vi "Sort CSV Array.vi"(10 "ListBox Tests in":T1, 11 "New ItemNames":string[](array[string])) -> (2 "Sorted ListBox Tests":T1)   [LabVIEW 2011]
uses:
  Controls/ListBox Test Record.ctl
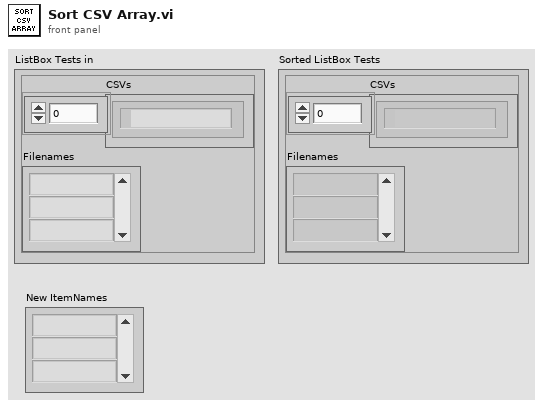
[diagram p1: front panel]
types:
  T1 = typedef "ListBox Test Record.ctl" = cluster{"CSVs":path[], "Filenames":string[]}
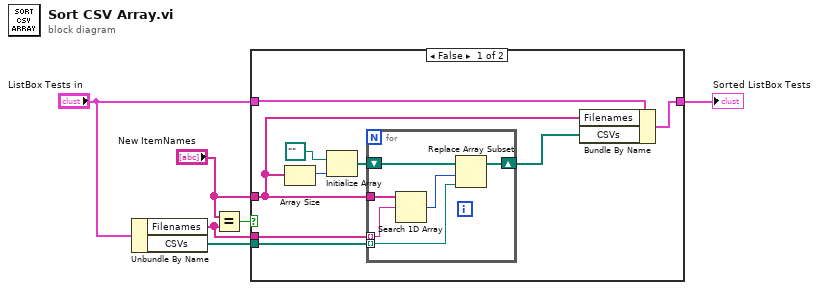
[diagram p0: block diagram]
diagram:
  n1 = Unbundle By Name("ListBox Tests in") -> ("Filenames"=w3:string[], "CSVs"=w1:path[])
  n2 = Equal?(x="New ItemNames", y=w3) -> (x = y?=w6:bool)
  n3 = case shown="False" w6 {
    tunnel: [w8 w22] -> w5
    tunnel: "ListBox Tests in" -> [w10 w22]
    tunnel: w3 -> [w15 _]
    tunnel: "New ItemNames" -> [w7 _]
    tunnel: w1 -> [w11 _]
    frame False {
      n4 = Array Size(array=w7) -> (size(s)=w14:i32)
      n5 = Initialize Array(path "", w14) -> (w12:path[])
      n6 = for {
        tunnel: w15 -> [w20] mode=indexing
        tunnel: w7 -> [w21]
        shift-right: [w16] -> w9
        shift-left: w12 -> [w19]
        tunnel: w11 -> [w18] mode=indexing
        n7 = Search 1D Array(1D array=w21, element=w20) -> (index of element=w17:i32)  [unwired: 1 in]
        n8 = Replace Array Subset(array=w19, new element=w18, index=w17) -> (w16:path[])
      }
      n9 = Bundle By Name(cluster=w10, "Filenames"=w7, "CSVs"=w9) -> (w8:T1)
    }
    frame True {
    }
  }
  "Sorted ListBox Tests" <- w5
